vi "Timeout.vi"(8 "Error In":errorcluster, 9 "TimeoutName":string, 10 "TimeoutID":u32, 11 "reference in":refnum<class "TimedDoor2.lvclass">) -> (0 "Error Out":errorcluster, 3 "reference in":refnum<class "TimedDoor2.lvclass">)   [LabVIEW 2020, in "TimedDoor2.lvclass"]
uses:
  TimedDoor2.lvclass
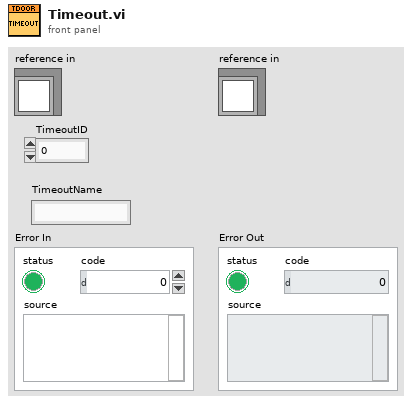
[diagram p1: front panel]
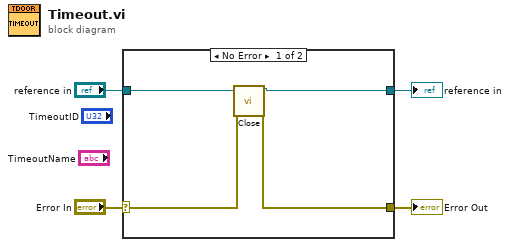
[diagram p0: block diagram]
diagram:
  n1 = case shown="No Error" "Error In" {
    selector: "Error In" -> [w8 w10]
    tunnel: [w7 w10] -> w3
    tunnel: [w5 w9] -> w1
    tunnel: "reference in" -> [w6 w9]
    frame No Error {
      n2 = call-dynamic "Close.vi"("reference in"=w6, "error in (no error)"=w8) -> ("reference out"=w5:refnum<class "TimedDoor2.lvclass">, "error out"=w7:errorcluster)  [unwired: 16 in]
    }
    frame Error {
    }
  }
  "Error Out" <- w3
  "reference in" <- w1
